vi "LV8_2.vi"() -> ()   [LabVIEW 2016]
uses:
  <vilib>/imath/engines/lvmath2/RunTimeEngine/BuiltInFunctions/linramp/NIMS_linramp.vi
  <vilib>/imath/engines/lvmath2/RunTimeEngine/BuiltInFunctions/polyval/NIMS_polyval(GV,GM).vi
  <instcachedir>/0/NIMS_polyval(GV,GM)_E12556DC54744E0C81968744501C4F35.lvgen/NIMS_polyval(GV,GM)_E12556DC54744E0C81968744501C4F35_003.vi
  <vilib>/imath/engines/lvmath2/RunTimeEngine/ArithmeticOperatorToken/NIMS_ArithmeticOperator_rightdiv(C,C).vi
  <instcachedir>/0/NIMS_ArithmeticOperator_rightdiv(C,C)_6F3C2C239EC94040B0793F3E73F9E5CA.lvgen/NIMS_ArithmeticOperator_rightdiv(C,C)_6F3C2C239EC94040B0793F3E73F9E5CA_000.vi
  <vilib>/imathl/engines/lvmath/Functions/Error Handling/Create Error.vi
  <vilib>/imath/engines/lvmath2/RunTimeEngine/BuiltInFunctions/filter/NIMS_filter(GV,GV,GV,GV,Str).vi
  <instcachedir>/0/NIMS_filter(GV,GV,GV,GV,Str)_434E59EE96884CB3BC5141C85D3A0B2F.lvgen/NIMS_filter(GV,GV,GV,GV,Str)_434E59EE96884CB3BC5141C85D3A0B2F_000.vi
  <vilib>/imath/engines/lvmath2/RunTimeEngine/BuiltInFunctions/fft/NIMS_fft(GV).vi
  <instcachedir>/0/NIMS_fft(GV)_4C6467FC22F84E4BA42517A07EF978B0.lvgen/NIMS_fft(GV)_4C6467FC22F84E4BA42517A07EF978B0_000.vi
  <vilib>/imath/engines/lvmath2/RunTimeEngine/BuiltInFunctions/fftshift/NIMS_fftshift(GV).vi
  <instcachedir>/0/NIMS_fftshift(GV)_BD7A7BA9CA6B470B9A9F73A6A3FEEB3E.lvgen/NIMS_fftshift(GV)_BD7A7BA9CA6B470B9A9F73A6A3FEEB3E_000.vi
  <vilib>/imath/engines/lvmath2/RunTimeEngine/BuiltInFunctions/abs/NIMS_abs(signed).vi
  <instcachedir>/0/NIMS_abs(signed)_C4FCB8E6058B49B797C7C8D53CA5F6EC.lvgen/NIMS_abs(signed)_C4FCB8E6058B49B797C7C8D53CA5F6EC_006.vi
  <vilib>/imath/engines/lvmath2/RunTimeEngine/ErrorHandling/NIMS_Error From Error Code.vi
  <vilib>/imath/engines/lvmath2/RunTimeEngine/NodeEndStatement/NIMS_NodeEndStatement_Output.vi
  <instcachedir>/0/NIMS_NodeEndStatement_Output_53EC0D466D134D7ABD903AC30B43404B.lvgen/NIMS_NodeEndStatement_Output_53EC0D466D134D7ABD903AC30B43404B_005.vi
  <instcachedir>/0/NIMS_NodeEndStatement_Output_53EC0D466D134D7ABD903AC30B43404B.lvgen/NIMS_NodeEndStatement_Output_53EC0D466D134D7ABD903AC30B43404B_000.vi
  <instcachedir>/0/NIMS_NodeEndStatement_Output_53EC0D466D134D7ABD903AC30B43404B.lvgen/NIMS_NodeEndStatement_Output_53EC0D466D134D7ABD903AC30B43404B_004.vi
  <vilib>/imath/engines/lvmath2/RunTimeEngine/ErrorHandling/NIMS_Finalize Error.vi
panel:
  out "Pole-Zero Plot":cluster{dbl[], dbl[]}[](graph)=[{array[401 elements], array[401 elements]}, {[0.3090169943749475, 0.3090169943749475], [-0.9510565162951535, 0.9510565162951535]}, {[0.2781152949374528, 0.2781152949374528], [0.8559508646656382, -0.8559508646656382]}]
  in  "notch frequency":dbl(slide)=200.0 scale=100.0..300.0
  in  "pole radius":dbl(slide)=0.9 scale=0.5..0.99
  in  "f2":dbl(slide)=200.0 scale=100.0..300.0
  in  "f1":dbl(slide)=125.0 scale=100.0..300.0
  out "Filtered (freq domain)":cluster{"W":dbl[], "FY":dbl[]}(graph)
  out "Signal (time domain)":cluster{"N":i32[], "X":dbl[]}(graph)={"N"=[1, 2, 3, 4, 5, 6, 7, 8, 9, 10, 11, 12, 13, 14, 15, 16, 17, 18, 19, 20, 21, 22, 23, 24, 25, 26, 27, 28, 29, 30, 31, 32, 33, 34, 35, 36, 37, 38, 39, 40, 41, 42, 43, 44, 45, 46, 47, 48, 49, 50], "X"=[1.658163297481701, 1.5877852522924734, 0.11932152889407455, -0.9510565162951535, -0.7071067811865477, -0.04894348370484647, -0.11932152889407432, -0.587785252292473, -0.2439497351086064, 0.9999999999999996, 1.6581632974817018, 0.5877852522924739, -1.2948920334790204, -1.9510565162951536, -0.7071067811865492, 0.9510565162951529, 1.2948920334790217, 0.41221474770752753, -0.2439497351086053, -3.6739403974420594e-16, 0.24394973510860563, -0.412214747707526, -1.2948920334790208, -0.9510565162951548, 0.7071067811865464, 1.9510565162951532, 1.294892033479023, -0.5877852522924711, -1.6581632974817015, -1.0000000000000016, 0.2439497351086043, 0.5877852522924734, 0.11932152889407566, 0.048943483704845914, 0.7071067811865472, 0.9510565162951541, -0.11932152889407277, -1.5877852522924716, -1.6581632974817033, -3.1840816777831186e-15, 1.6581632974816978, 1.5877852522924747, 0.11932152889407766, -0.9510565162951493, -0.7071067811865493, -0.048943483704847135, -0.11932152889407166, -0.5877852522924727, -0.24394973510860973, 0.9999999999999976]}
  out "Original signal (freq domain)":cluster{"W":dbl[], "H":dbl[]}[](graph)
  out "Filtered signal (time domain)":cluster{"N":i32[], "Y":dbl[]}(graph)={"N"=[1, 2, 3, 4, 5, 6, 7, 8, 9, 10, 11, 12, 13, 14, 15, 16, 17, 18, 19, 20, 21, 22, 23, 24, 25, 26, 27, 28, 29, 30, 31, 32, 33, 34, 35, 36, 37, 38, 39, 40, 41, 42, 43, 44, 45, 46, 47, 48, 49, 50], "Y"=[1.658163297481701, 1.485305124618344, 0.2792394482737034, -0.48479165236005406, -0.49583989986036237, -0.4461040571223799, -0.6426859775750758, -0.5591212896929659, 0.2095752770582735, 1.1324444001838025, 1.2563238159207697, 0.3445097486058005, -0.8259954302111623, -1.3014807973022087, -0.8510467067464296, 0.017837258558947244, 0.6992694613145982, 0.9374908610669572, 0.7512324046119836, 0.22147482163740884, -0.485307177053892, -1.0123212784406914, -0.9661648220595325, -0.28041416890477666, 0.6266185672890349, 1.1386638676737966, 0.9219782089045203, 0.1534987257261733, -0.6614216624569447, -1.0552209048538448, -0.8473741733882614, -0.17959047892807822, 0.5864793624144107, 1.0346700251881493, 0.896646408503817, 0.2236434158600713, -0.6018862817626024, -1.0789227039402605, -0.9087814974376135, -0.1945486537466914, 0.6278991004915758, 1.0698250721343487, 0.8826507331612748, 0.18738300508217437, -0.6107189344112437, -1.0544647628030759, -0.8880227937663492, -0.2028129600797074, 0.6064876905313316, 1.064609479071854]}
  in  "stop":bool
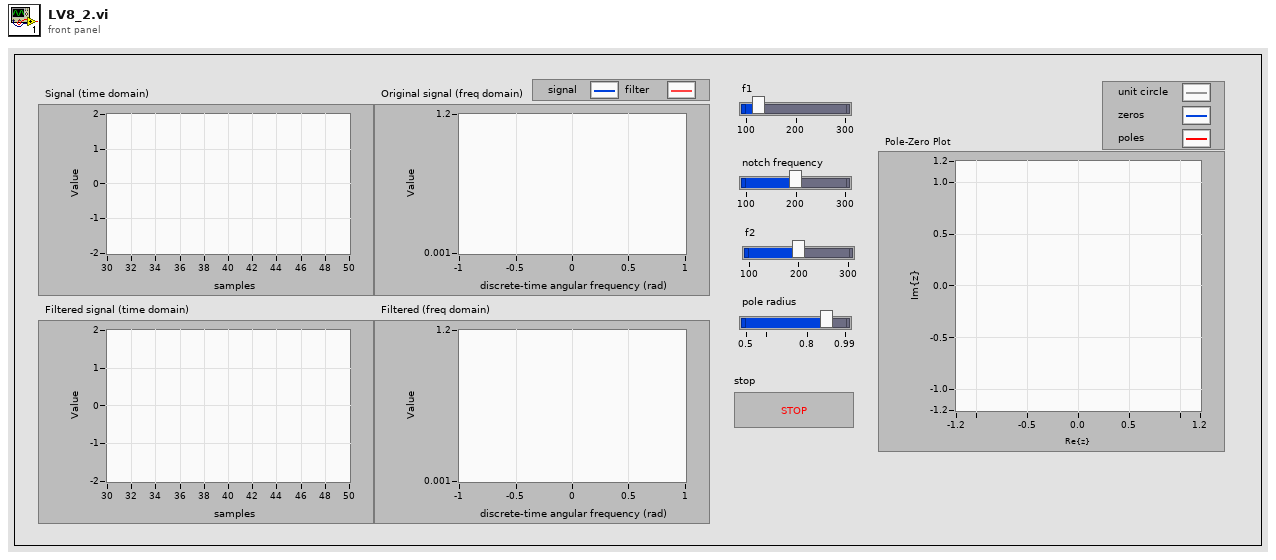
[diagram p1: front panel]
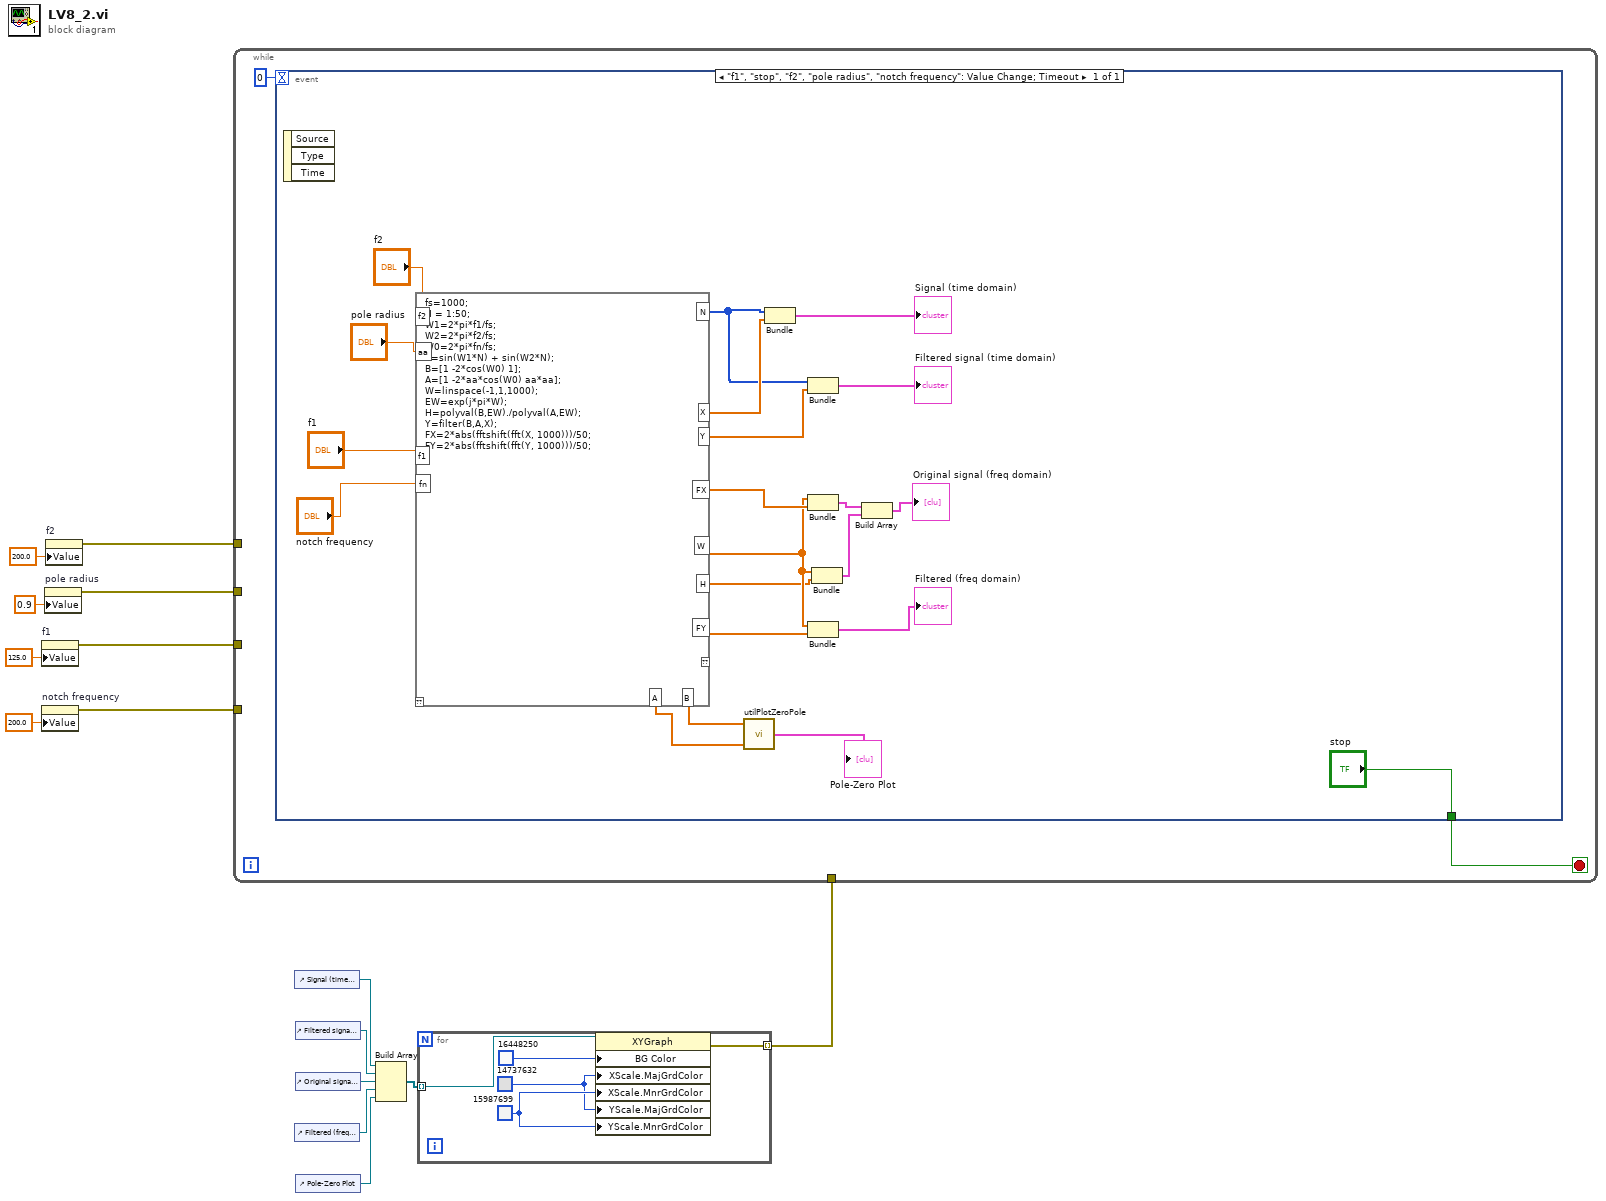
[diagram p0: block diagram]
diagram:
  n1 = property on="f1" class="Slide (strict)"("Value"=125.0 ("Interference level")) -> (error out=w13:errorcluster)  [unwired: 2 in, 1 out]
  n2 = property on="notch frequency" class="Slide (strict)"("Value"=200.0 ("notch frequency")) -> (error out=w9:errorcluster)  [unwired: 2 in, 1 out]
  n3 = property on="pole radius" class="Slide (strict)"("Value"=0.9 ("pole radius")) -> (error out=w14:errorcluster)  [unwired: 2 in, 1 out]
  n4 = property on="f2" class="Slide (strict)"("Value"=200.0 ("Interference frequency")) -> (error out=w15:errorcluster)  [unwired: 2 in, 1 out]
  n5 = control-ref of="Signal (time domain)"() -> (w5:refnum<vi>)
  n6 = control-ref of="Filtered (freq domain)"() -> (w2:refnum<vi>)
  n7 = control-ref of="Filtered signal (time domain)"() -> (w4:refnum<vi>)
  n8 = control-ref of="Original signal (freq domain)"() -> (w3:refnum<vi>)
  n9 = control-ref of="Pole-Zero Plot"() -> (w1:refnum<vi>)
  n10 = Build Array(w5, w4, w3, w2, w1) -> (w7:refnum<vi>[])
  n11 = for {
    tunnel: w7 -> [w17] mode=indexing
    tunnel: [w16] -> w6 mode=indexing
    w19 = u32 15987699
    w18 = u32 14737632
    n12 = property class="XYGraph"(reference=w17, "BG Color"=u32 16448250, "XScale.MajGrdColor"=w18, "XScale.MnrGrdColor"=w19, "YScale.MajGrdColor"=w18, "YScale.MnrGrdColor"=w19) -> (error out=w16:errorcluster)  [unwired: 1 in, 1 out]
  }
  n13 = while {
    tunnel: w15 -> [_]
    tunnel: w14 -> [_]
    tunnel: w13 -> [_]
    tunnel: w9 -> [_]
    tunnel: w6 -> [_]
    stop <- w22 stop-if-true
    n14 = event shown="[0] \"f1\", \"stop\", \"f2\", \"pole radius\", \"notch frequency\": Value Change;  Timeout" {
      selector: _ -> [_]
      dyn-events: _ -> [_]
      timeout: 0 -> [_]
      tunnel: ["stop"] -> w22
      event "f1", "stop", "f2", "pole radius", "notch frequency": Value Change; Timeout {
        n15 = event-data() -> ()  [unwired: 1 in, 3 out]
        n16 = mathscript code="fs=1000;\nN = 1:50;\nW1=2*pi*f1/fs;\nW2=2*pi*f2/fs;\nW0=2*pi*fn/fs;\nX=sin(W1*N) + sin(W2*N);\nB=[1 -2*cos(W0) 1];\nA=[1 -2*aa*cos(W0) aa*aa];\nW=linspace(-1,1,1000);\nEW=exp(j*pi*W);\nH=polyval(B,EW)./polyval(A,EW);\nY=filter(B,A,X);\nFX=2*abs(fftshift(fft(X, 1000)))/50;\nFY=2*abs(fftshift(fft(Y, 1000)))/50;"("aa"="pole radius", "f1"="f1", "f2"="f2", "fn"="notch frequency") -> ("Y"=w40:dbl[], "X"=w41:dbl[], "W"=w36:dbl[], "FY"=w38:dbl[], "N"=w31:i32[], "FX"=w37:dbl[], "H"=w32:cdb[], "B"=w24:dbl[], "A"=w23:dbl[])  [unwired: 1 in, 1 out]
        n17 = call "utilPlotZeroPole.vi"("a, reverse coefficients"=w23, "b, forward coefficients"=w24) -> ("Pole-Zero Plot"=→"Pole-Zero Plot":cluster{dbl[], dbl[]}[])  [unwired: 3 in]
        n18 = Bundle("N"=w31, "X"=w41) -> (→"Signal (time domain)":cluster{"N":i32[], "X":dbl[]})  [unwired: 1 in]
        n19 = Bundle("N"=w31, "Y"=w40) -> (→"Filtered signal (time domain)":cluster{"N":i32[], "Y":dbl[]})  [unwired: 1 in]
        n20 = Bundle("W"=w36, "FX"=w37) -> (w28:cluster{"W":dbl[], "FX":dbl[]})  [unwired: 1 in]
        n21 = Bundle("W"=w36, "FY"=w38) -> (→"Filtered (freq domain)":cluster{"W":dbl[], "FY":dbl[]})  [unwired: 1 in]
        n22 = Bundle("W"=w36, "H"=w32) -> (w29:cluster{"W":dbl[], "H":cdb[]})  [unwired: 1 in]
        n23 = Build Array(w28, w29) -> (→"Original signal (freq domain)":cluster{"W":dbl[], "H":cdb[]}[])
      }
    }
  }
